vi "Start Sync.vi"(8 "error in (no error)":errorcluster, 11 "gRPC Server in":refnum<class "Temperature_server.lvclass">) -> (0 "error out":errorcluster, 3 "gRPC Server out":refnum<class "Temperature_server.lvclass">)   [LabVIEW 2019, in "Temperature_server.lvlib" / "Temperature_server.lvclass"]
uses:
  Temperature_server.lvclass
  Temperature_server.lvclass/Temperature_server.ctl
  TemperatureSensor/TemperatureSensor.lvclass
  RPC Messages/Temperature/Temperature_Data.ctl
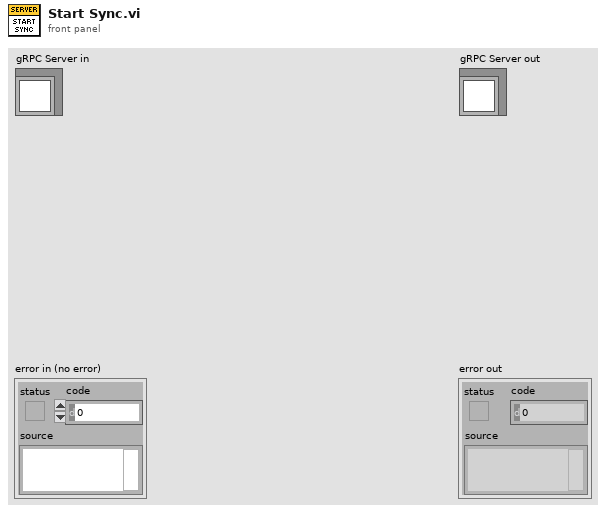
[diagram p1: front panel]
types:
  T1 = typedef "Temperature_server.lvlib/Temperature_server.lvclass/Temperature_Data.ctl" = cluster{"temperature":dbl}
  T2 = typedef "Temperature_server.lvlib/Temperature_server.lvclass/Server gRPC UEs.ctl" = cluster{"TemperatureService_MethodName gRPC UE":refnum<user-event>}
  T3 = typedef "gprc-lvsupport-release.lvlib/grpcId.ctl" = u64
  T4 = typedef "Temperature_server.lvlib/Temperature_server.lvclass/Units_Data.ctl" = cluster{"unit":i32}
  T5 = typedef "Temperature_server.lvlib/Temperature_server.lvclass/Server State Data.ctl" = cluster{"TemperatureSensor":refnum<class "TemperatureSensor.lvclass">}
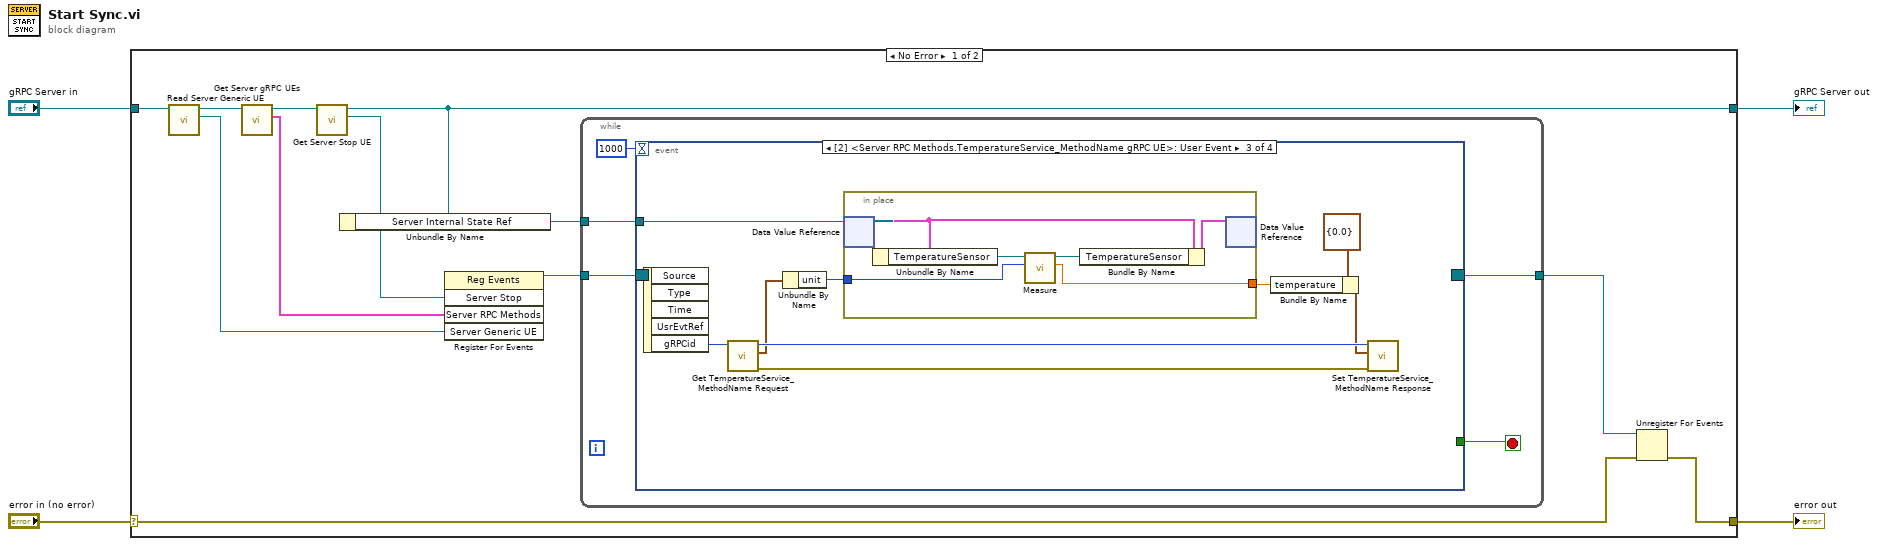
[diagram p0: block diagram]
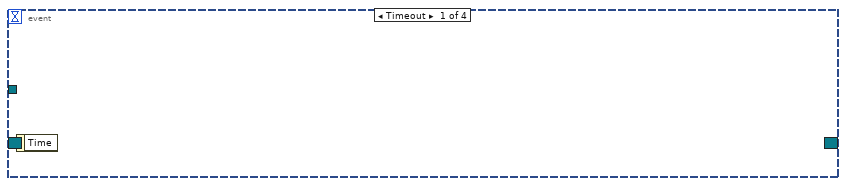
[diagram p2: hidden frame]
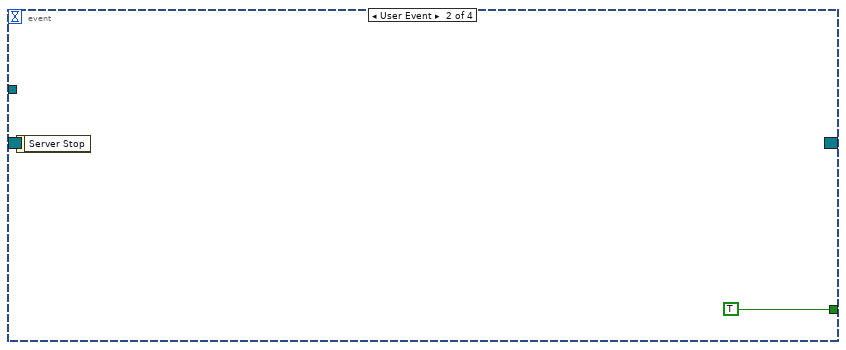
[diagram p3: hidden frame]
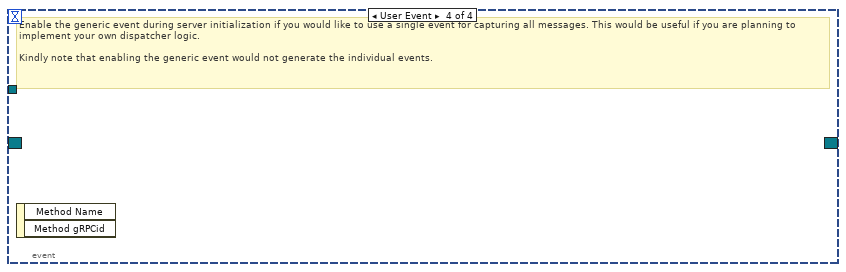
[diagram p4: hidden frame]
diagram:
  n1 = case shown="No Error" "error in (no error)" {
    selector: "error in (no error)" -> [w11 w39]
    tunnel: [w10 w39] -> w3
    tunnel: [w6 w38] -> w1
    tunnel: "gRPC Server in" -> [w9 w38]
    frame No Error {
      n2 = call "Read Server Generic UE.vi"("Template Server in"=w9) -> ("Server Generic UE"=w7:refnum<user-event>, "Template Server out"=w8:refnum<class "Temperature_server.lvclass">)  [unwired: 9 in]
      n3 = call "Get Server gRPC UEs.vi"("OOP Server in"=w8) -> ("Server RPC Methods"=w14:T2, "OOP Server out"=w16:refnum<class "Temperature_server.lvclass">)  [unwired: 9 in]
      n4 = call "Get Server Stop UE.vi"("OOP Server in"=w16) -> ("Server Stop"=w15:refnum<user-event>, "OOP Server out"=w6:refnum<class "Temperature_server.lvclass">)  [unwired: 9 in]
      n5 = Unbundle By Name(w6) -> ("Server Internal State Ref"=w5:refnum<data-value>)
      n6 = register-events(w15, w14, w7) -> (reference out=w13:refnum<event-registration>)  [unwired: 2 in, 1 out]
      n7 = while {
        tunnel: w13 -> [w21]
        tunnel: [w19] -> w12
        tunnel: w5 -> [w17]
        stop <- w20 stop-if-true
        n8 = event "RPC Methods Event Structure" shown="[2] <Server RPC Methods.TemperatureService_MethodName gRPC UE>: User Event" {
          selector: w21 -> [_ _ _ _]
          dyn-events: [_ _ _ _] -> w19
          timeout: 1000 -> [_ _ _ _]
          tunnel: [_ TRUE _ _] -> w20
          tunnel: w17 -> [_ _ w28 _]
          event Timeout {
            n9 = event-data() -> ()  [unwired: 1 in, 1 out]
          }
          event User Event {
            n10 = event-data() -> ()  [unwired: 1 in, 1 out]
          }
          event User Event {
            n11 = event-data() -> ("gRPCid"=w31:T3)  [unwired: 1 in, 4 out]
            n12 = call "Get TemperatureService_MethodName Request.vi"("gRPCid in"=w31) -> ("error out"=w23:errorcluster, "Message Data"=w29:T4, "gRPCid out"=w30:T3)  [unwired: 8 in]
            n13 = Unbundle By Name(w29) -> ("unit"=w27:i32)
            n14 = in-place {
              in-place-border: w27 -> [w33]
              in-place-border: [w32] -> w24
              n15 = in-place-dvr #1(w28) -> (w36:T5)  [unwired: 1 out]
              n16 = Unbundle By Name(w36) -> ("TemperatureSensor"=w37:refnum<class "TemperatureSensor.lvclass">)
              n17 = call "Measure.vi"("unit"=w33, "TemperatureSensor in"=w37) -> ("measurement"=w32:dbl, "TemperatureSensor out"=w34:refnum<class "TemperatureSensor.lvclass">)  [unwired: 7 in, 1 out]
              n18 = Bundle By Name(cluster=w36, "TemperatureSensor"=w34) -> (w35:T5)
              n19 = in-place-dvr #1(w35) -> ()  [unwired: 2 out]
            }
            n20 = Bundle By Name(cluster=T1 {"temperature"=0.0} ("Message Data"), "temperature"=w24) -> (w25:T1)
            n21 = call "Set TemperatureService_MethodName Response.vi"("error in (no error)"=w23, "Message Data"=w25, "gRPCid in"=w30) -> ()  [unwired: 8 in, 1 out]
          }
          event User Event {
            # "Enable the generic event during server initialization if you would like to use a single event for capturing all messages. This would be useful if you are planning to implement your own dispatcher logic. \n\nKindly note that enabling the generic event would not generate the individual events."
            n22 = event-data() -> ()  [unwired: 1 in, 2 out]
          }
        }
      }
      n23 = Unregister For Events(event registration refnum=w12, error in=w11) -> (error out=w10:errorcluster)
    }
    frame Error {
    }
  }
  "error out" <- w3
  "gRPC Server out" <- w1
